vi "Vision Research Phantom Series PhFile PhfReduceDIB16To8.vi"(0 "BITMAPINFOHEADER":T2, 1 "PRANGE":T1, 2 "pPixel16 in":u16[](array[numeric]), 5 "Error In (no error)":errorcluster) -> (16 "pPixel8 out":u8[](array[numeric]), 19 "Error Out":errorcluster)   [LabVIEW 2013, in "VRI.lvlib"]
doc: "PhFile.dll\n\nPhfReduceDIB16To8\nvoid PhfReduceDIB16To8(PBITMAPINFOHEADER pBMIH, PRANGE pPixRng, PWORD pPixel16, PBYTE pPixel8);\n\nParameters Description\npBMIH(in) Pointer to BITMAPINFOHEADER structure that corresponds to the \n cine images.\npPixRng(in) Image range (first image and count)\npPixel16(in) 16-bit Image Pixels\npPixel8(out) 8-bit Image Pixels\nReturn void\nComments Converts an array of 16-bit image pixels into an array of 8-bit \n image pixels."
uses:
  VRI.lvlib
  _Type Defs/BITMAPINFOHEADER.ctl
  _Type Defs/PhFile PRANGE.ctl
  Phantom DLLs/PhFile.Dll
panel:
  # "For instructions on the use of this VI, press Ctrl+H to display the help window and move the mouse over the icon, controls, and indicators"
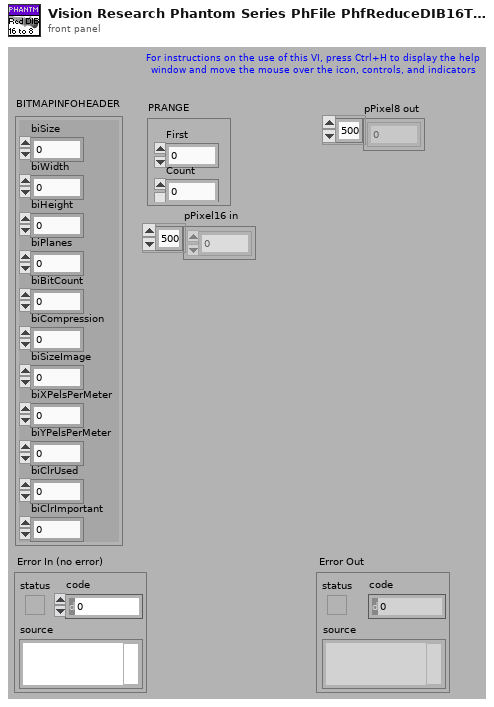
[diagram p1: front panel]
types:
  T1 = typedef "VRI.lvlib/PhFile PRANGE.ctl" = cluster{"First":u32, "Count":u32}
  T2 = typedef "VRI.lvlib/BITMAPINFOHEADER.ctl" = cluster{"biSize":u32, "biWidth":i32, "biHeight":i32, "biPlanes":u16, "biBitCount":u16, "biCompression":u32, "biSizeImage":u32, "biXPelsPerMeter":i32, "biYPelsPerMeter":i32, "biClrUsed":u32, "biClrImportant":u32}
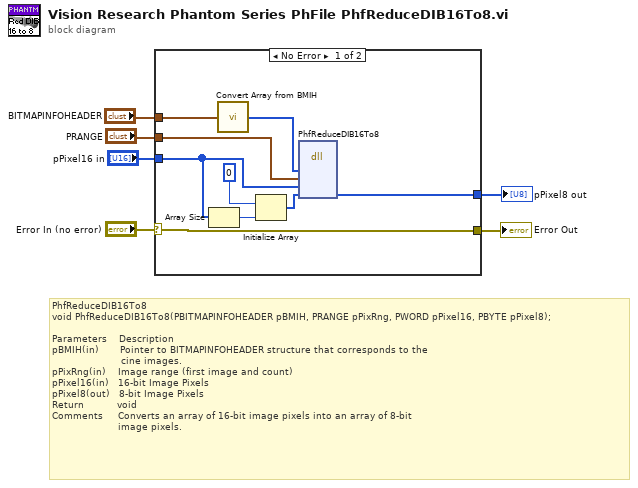
[diagram p0: block diagram]
diagram:
  # "PhfReduceDIB16To8\nvoid PhfReduceDIB16To8(PBITMAPINFOHEADER pBMIH, PRANGE pPixRng, PWORD pPixel16, PBYTE pPixel8);\n\nParameters    Description\npBMIH(in)       Pointer to BITMAPINFOHEADER structure that corresponds to the \n                       cine images.\npPixRng(in)    Image range (first image and count)\npPixel16(in)   16-bit Image Pixels\npPixel8(out)   8-bit Image Pixels\nReturn           void\nComments     Converts an array of 16-bit image pixels into an array of 8-bit \n                      image pixels."
  n1 = case shown="No Error" "Error In (no error)" {
    selector: "Error In (no error)" -> [w15 w16]
    tunnel: [w15 w16] -> w5
    tunnel: "BITMAPINFOHEADER" -> [w14 _]
    tunnel: "PRANGE" -> [w13 _]
    tunnel: "pPixel16 in" -> [w12 _]
    tunnel: [w11 _] -> w3
    frame No Error {
      n2 = Array Size(array=w12) -> (size(s)=w8:i32)
      n3 = call "Convert Array from BMIH.vi"("BITMAPINFOHEADER"=w14) -> ("Array"=w10:u8[])
      n4 = Initialize Array(u8 0, w8) -> (w7:u8[])
      n5 = dll-call lib="C:/Projects/SDK/64-bit/Vision Research Phantom Series Labview Driver/Phantom DLLs/PhFile.dll" fn="PhfReduceDIB16To8"("pBMIH"=w10, "pPixRng"=w13, "pPixel16"=w12, "pPixel8"=w7) -> ("pPixel8"=w11:u8[])  [unwired: 6 in, 3 out]
    }
    frame Error {
    }
  }
  "Error Out" <- w5
  "pPixel8 out" <- w3
